vi "Pulse and Trigger Generation.vi"() -> ()   [LabVIEW 2026]
uses:
  <vilib>/Platform/TimedLoop/XDataNode/timing_clust.ctl
  <vilib>/Platform/TimedLoop/XDataNode/nitl_modes.ctl
  <vilib>/Platform/TimedLoop/XDataNode/wakeup.ctl
  <vilib>/rvi/Emulation/niFpgaGetClockAttributes.vi
  <vilib>/rvi/Emulation/niFpgaSctlEmulationGetInTimedLoop.vi
  <vilib>/rvi/Emulation/niFpgaEmulationReportErrorSimple.vi
  <vilib>/rvi/Emulation/niFpgaProcessEmulError.vi
  <vilib>/rvi/Emulation/niFpgaCriticalErrorInLSC.vi
  <vilib>/rvi/eio/common/nirviEmuTemplateMethod_errors.vi
  <vilib>/platform/TimedLoop/XDataNode/XDataNode.xnode
  <vilib>/eio/EIONode/EIONode.xnode
  <vilib>/Platform/TimedLoop/XDataNode/XDNodeRunTimeDep.lvlib
panel:
  in  "Trigger":bool
  out "Output":bool
  in  "Enable Output":bool
  out "Requested Output Ticks":i32
  in  "Requested Output Frequency":sgl
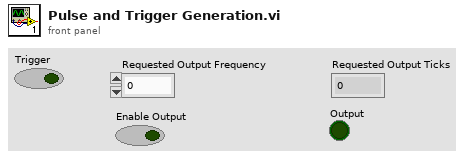
[diagram p1: front panel]
types:
  T1 = typedef "XDNodeRunTimeDep.lvlib/timing_clust.ctl" = cluster{"Expected End [f-1]":u64, "Actual End [f-1]":u64, "Finished Late? [f-1]":bool, "Expected End [i-1]":u64, "Actual End [i-1]":u64, "Finished Late? [i-1]":bool, "Expected Start [i]":u64, "Actual Start [i]":u64, "Expected Start [f]":u64, "Actual Start [f]":u64, "Source Name":string, "Structure Name":string, "Period":i64, "Deadline":i64, "Offset":i64, "Start":i64, "Priority":i32, "Timeout":i32, "Mode":T2, "Wakeup Reason":T3, "Error":errorcluster, "Source Type":string, "Secondary Source Type":string, "Global End Time":u64, "Global Start Time":u64, "Frame Duration":u64, "Iteration Duration":u64, "Assigned CPU":i32, "I/O Scan Engine Mode":u32}
  T2 = typedef "XDNodeRunTimeDep.lvlib/nitl_modes.ctl" = enum32{"No Change", "Process missed periods, maintain original phase", "Discard missed periods, maintain original phase", "Process missed periods, ignore original phase", "Discard missed periods, ignore original phase"}
  T3 = typedef "XDNodeRunTimeDep.lvlib/wakeup.ctl" = enum32{"Normal", "Aborted", "Asynchronous wakeup", "Timing source error", "Timed loop error", "Timeout"}
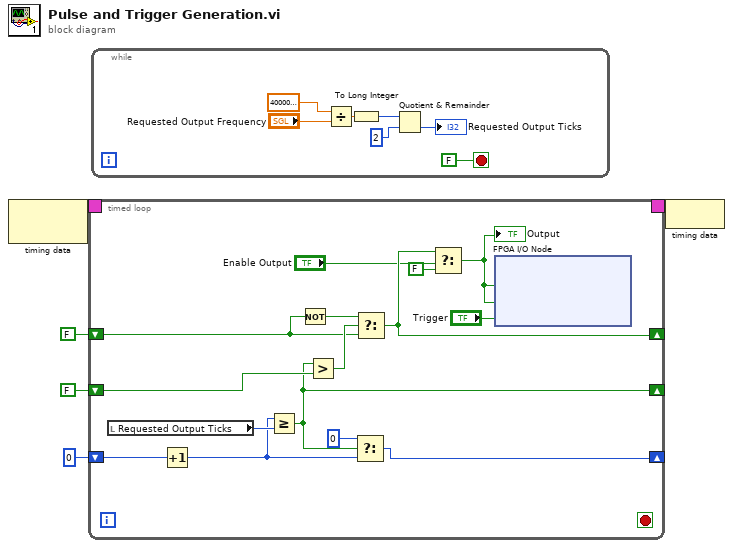
[diagram p0: block diagram]
diagram:
  n1 = node-c288() -> (w5:T1)  [unwired: 1 in]
  n2 = timed-loop {
    timing: w5 -> [_]
    timing-out: [_] -> w4
    shift-right: [w20] -> _
    shift-left: 0 -> [w19]
    shift-right: [w15] -> _
    shift-left: FALSE -> [w16]
    shift-right: [w9] -> _
    shift-left: FALSE -> [w13]
    stop <- _ stop-if-true
    n3 = local read "Requested Output Ticks"() -> (w18:i32)
    n4 = Increment(x=w19) -> (x+1=w11:i32)
    n5 = Greater Or Equal?(x=w11, y=w18) -> (x >= y?=w15:bool)
    n6 = Not(x=w13) -> (.not. x?=w12:bool)
    n7 = Greater?(x=w15, y=w16) -> (0:w14:bool)
    n8 = Select(t=0, s=w15, f=w11) -> (s? t:f=w20:i32)
    n9 = Select(t=w12, s=w14, f=w13) -> (s? t:f=w9:bool)
    n10 = Select(t=w9, s="Enable Output", f=FALSE) -> (s? t:f=w7:bool)
    "Output" <- w7
    n11 = xnode "FPGA I/O Node"("Connector1/DIO0"=w7, "Connector1/DIO1"=w7, "Connector1/DIO2"="Trigger") -> ()  [unwired: 3 in, 3 out]
  }
  n12 = while {
    stop <- FALSE stop-if-true
    n13 = Divide(x=sgl 40000000.0 ("y"), y="Requested Output Frequency") -> (x/y=w27:sgl)
    n14 = To Long Integer(number=w27) -> (32bit integer=w24:i32)
    n15 = Quotient & Remainder(x=w24, y=2) -> (floor(x/y)=→"Requested Output Ticks":i32)  [unwired: 1 out]
  }
  n16 = node-c288(w4) -> ()
